vi "Do Turn.vi"(11 "SB App in":refnum<class "SB App.lvclass">) -> (3 "SB App out":refnum<class "SB App.lvclass">)   [LabVIEW 2020, in "SB App.lvlib" / "SB App.lvclass"]
uses:
  SB App.lvclass
  SB App.lvclass/SB App.ctl
  SquareBattle/Game/Game.lvclass/Game.ctl
  SquareBattle/Map/Map.lvclass/Map.ctl
  SquareBattle/Game/Game.lvclass
  Square Field Panel/Square Field Panel.lvclass
  Team Field Panel/Team Field Panel.lvclass
  Dashboard Panel/Dashboard Panel.lvclass
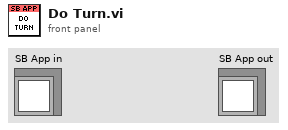
[diagram p1: front panel]
types:
  T1 = typedef "SB App.lvlib/Display Mode.ctl" = enum16{"Config", "Team", "Squares", "Done"}
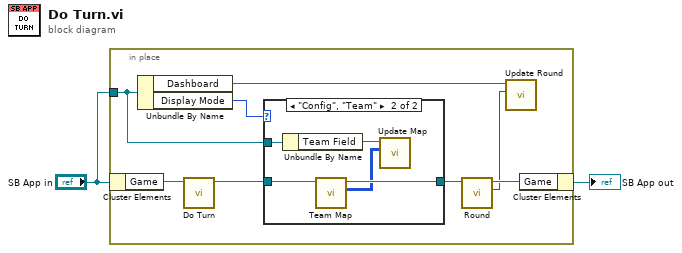
[diagram p0: block diagram]
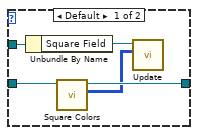
[diagram p2: hidden frame]
diagram:
  n1 = in-place {
    in-place-border: "SB App in" -> [w7]
    n2 = in-place-cluster #1("SB App in") -> ("Game"=w10:refnum<class "Game.lvclass">)
    n3 = Unbundle By Name(w7) -> ("Dashboard"=w4:refnum<class "Dashboard Panel.lvclass">, "Display Mode"=w8:T1)
    n4 = call "Do Turn.vi"("Game in"=w10) -> ("Game out"=w9:refnum<class "Game.lvclass">)  [unwired: 10 in]
    n5 = case shown="\"Config\", \"Team\"" w8 {
      tunnel: w9 -> [w15 w20]
      tunnel: [w14 w17] -> w6
      tunnel: w7 -> [w13 w19]
      frame Default {
        n6 = Unbundle By Name(w13) -> ("Square Field"=w12:refnum<class "Square Field Panel.lvclass">)
        n7 = call "Square Colors.vi"("Game in"=w15) -> ("Square Colors"=w11:u32[][], "Game out"=w14:refnum<class "Game.lvclass">)  [unwired: 9 in]
        n8 = call "Update.vi"("Square Colors"=w11, "Square Field Panel in"=w12) -> ()  [unwired: 8 in, 2 out]
      }
      frame "Config", "Team" {
        n9 = Unbundle By Name(w19) -> ("Team Field"=w18:refnum<class "Team Field Panel.lvclass">)
        n10 = call "Team Map.vi"("Game in"=w20) -> ("Team Map"=w16:i32[][], "Game out"=w17:refnum<class "Game.lvclass">)  [unwired: 9 in]
        n11 = call "Update Map.vi"("Team Map"=w16, "Team Field Panel in"=w18) -> ()  [unwired: 8 in, 2 out]
      }
    }
    n12 = call "Round.vi"("Game in"=w6) -> ("Round"=w3:u32, "Game out"=w5:refnum<class "Game.lvclass">)  [unwired: 8 in, 1 out]
    n13 = call "Update Round.vi"("Round"=w3, "Dashboard Panel in"=w4) -> ()  [unwired: 8 in, 2 out]
    n14 = in-place-cluster #1("Game"=w5) -> (→"SB App out":refnum<class "SB App.lvclass">)
  }
